vi "SPI Slave Continue Read.vi"(9 "pSlaveReadDataHandle":cluster{}, 10 "SPIIndex":i32, 11 "DevHandle":i32) -> (3 "function return":i32)   [LabVIEW 2010, in "usb2spi.lvlib"]
doc: "int WINAPI SPI_SlaveContinueRead(int DevHandle,int SPIIndex,PSPI_GET_DATA_HANDLE pSlaveReadDataHandle);"
uses:
  usb2spi.lvlib
  USB2XXX/trunk/USB2XXX/USB2XXX/vs2019/Release/USB2XXX.dll
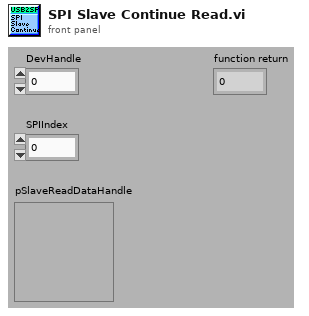
[diagram p1: front panel]
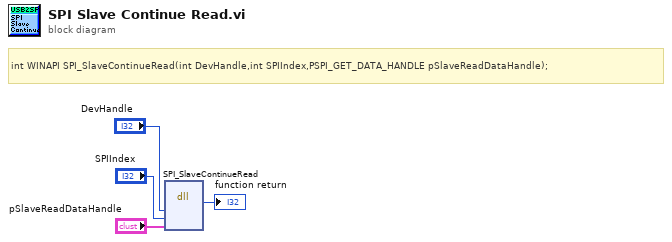
[diagram p0: block diagram]
diagram:
  # "int WINAPI SPI_SlaveContinueRead(int DevHandle,int SPIIndex,PSPI_GET_DATA_HANDLE pSlaveReadDataHandle);"
  n1 = dll-call lib="E:/Projects/USB2XXX/trunk/USB2XXX/USB2XXX/vs2019/Release/USB2XXX.*" fn="SPI_SlaveContinueRead"("DevHandle"="DevHandle", "SPIIndex"="SPIIndex", "pSlaveReadDataHandle"="pSlaveReadDataHandle") -> (→"function return":i32)  [unwired: 6 in, 2 out]
